vi "Message Loop Async.vi"(11 "OBS in":refnum<class "OBS.lvclass">) -> ()   [LabVIEW 2022 SP3, in "obs-websocket-lv.lvlib" / "OBS.lvclass"]
uses:
  OBS.lvclass
  State.ctl
  OBS.lvclass/OBS.ctl
  <vilib>/MediaMongrels Ltd/WebSockets/WebSockets/WebSocket Client/WebSocket Client.lvclass
panel:
  out "State":T1
  out "error IO":errorcluster
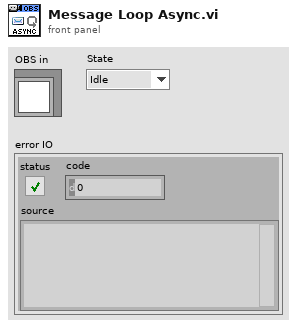
[diagram p1: front panel]
types:
  T1 = typedef "obs-websocket-lv.lvlib/OBS.lvclass/State.ctl" = enum16{"Idle", "Opening", "Open", "Closing", "Stopping"}
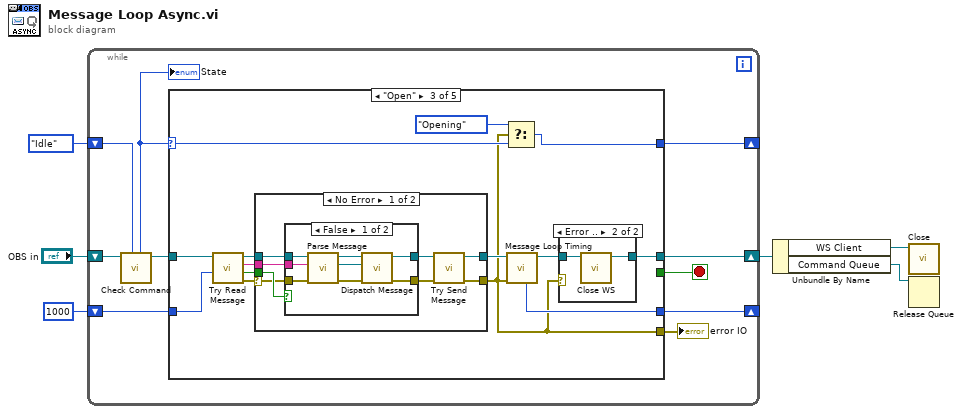
[diagram p0: block diagram]
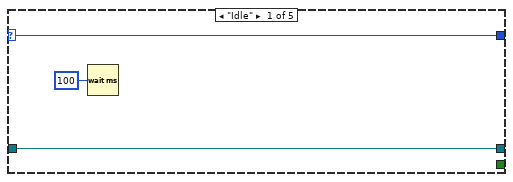
[diagram p2: hidden frame]
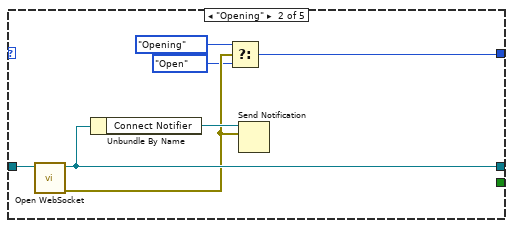
[diagram p3: hidden frame]
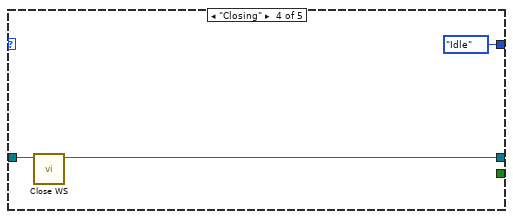
[diagram p7: hidden frame]
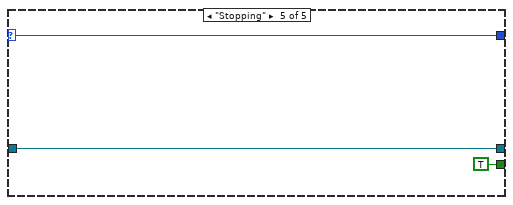
[diagram p8: hidden frame]
diagram:
  n1 = while {
    shift-right: [w12] -> _
    shift-left: 1000 -> [w13]
    shift-right: [w15] -> w5
    shift-left: "OBS in" -> [w11]
    shift-right: [w7] -> _
    shift-left: State."Idle" ("State") -> [w9]
    stop <- w16 stop-if-true
    n2 = call "Check Command.vi"("State"=w9, "OBS in"=w11) -> ("OBS out"=w10:refnum<class "OBS.lvclass">, "Next State"=w8:T1)  [unwired: 7 in, 1 out]
    "State" <- w8
    n3 = case shown="\"Open\"" w8 {
      selector: w8 -> [w18 _ w32 _ w67]
      tunnel: w10 -> [w19 w26 w40 w65 w68]
      tunnel: [_ _ _ _ TRUE ("Stop?")] -> w16
      tunnel: [w19 w24 w27 w64 w68] -> w15
      tunnel: [_ _ w28 _ _] -> w14
      tunnel: w13 -> [_ _ w34 _ _]
      tunnel: [_ _ w33 _ _] -> w12
      tunnel: [w18 w20 w30 State."Idle" ("State") w67] -> w7
      frame "Idle" {
        n4 = Wait (ms)(milliseconds to wait=u32 100) -> ()  [unwired: 1 out]
      }
      frame "Opening" {
        n5 = call "Open WebSocket.vi"("OBS in"=w26) -> ("error out"=w23:errorcluster, "OBS out"=w24:refnum<class "OBS.lvclass">)  [unwired: 9 in]
        n6 = Unbundle By Name(w24) -> ("Connect Notifier"=w25:refnum<notifier>)
        n7 = Select(t=State."Opening" ("State"), s=w23, f=State."Open" ("State")) -> (s? t:f=w20:T1)
        n8 = Send Notification(notification=w23, notifier=w25) -> ()  [unwired: 1 in, 2 out]
      }
      frame "Open" {
        n9 = call "Try Read Message.vi"("timeout ms (100)"=w34, "OBS in"=w40) -> ("error out"=w39:errorcluster, "Timeout"=w38:bool, "Data"=w37:string, "OBS out"=w36:refnum<class "OBS.lvclass">)  [unwired: 6 in]
        n10 = case shown="No Error" w39 {
          selector: w39 -> [w50 w63]
          tunnel: w38 -> [w51 _]
          tunnel: w37 -> [w49 _]
          tunnel: w36 -> [w48 w62]
          tunnel: [w45 w62] -> w35
          tunnel: [w44 w63] -> w28
          frame No Error {
            n11 = case shown="False" w51 {
              tunnel: w50 -> [w57 w60]
              tunnel: w49 -> [w58 _]
              tunnel: w48 -> [w59 w61]
              tunnel: [w53 w61] -> w47
              tunnel: [w52 w60] -> w46
              frame False {
                n12 = call "Parse Message.vi"("error in (no error)"=w57, "Data"=w58, "OBS in"=w59) -> ("error out"=w54:errorcluster, "Server Message"=w55:refnum<class "Server Message.lvclass">, "OBS out"=w56:refnum<class "OBS.lvclass">)  [unwired: 6 in]
                n13 = call "Dispatch Message.vi"("error in (no error)"=w54, "Server Message"=w55, "OBS in"=w56) -> ("error out"=w52:errorcluster, "OBS out"=w53:refnum<class "OBS.lvclass">)  [unwired: 7 in]
              }
              frame True {
              }
            }
            n14 = call "Try Send Message.vi"("error in (no error)"=w46, "OBS in"=w47) -> ("error out"=w44:errorcluster, "OBS out"=w45:refnum<class "OBS.lvclass">)  [unwired: 8 in]
          }
          frame Error {
          }
        }
        n15 = Select(t=State."Opening", s=w28, f=w32) -> (s? t:f=w30:T1)
        n16 = call "Message Loop Timing.vi"("error in (no error)"=w28, "OBS in"=w35) -> ("OBS out"=w29:refnum<class "OBS.lvclass">, "Next Timeout"=w33:i32)  [unwired: 7 in, 1 out]
        n17 = case shown="Error .." w28 {
          tunnel: w29 -> [w41 w43]
          tunnel: [w41 w42] -> w27
          frame No Error {
          }
          frame Error {
            n18 = call "Close WS.vi"("OBS in"=w43) -> ("OBS out"=w42:refnum<class "OBS.lvclass">)  [unwired: 9 in, 1 out]
          }
        }
      }
      frame "Closing" {
        n19 = call "Close WS.vi"("OBS in"=w65) -> ("OBS out"=w64:refnum<class "OBS.lvclass">)  [unwired: 9 in, 1 out]
      }
      frame "Stopping" {
      }
    }
    "error IO" <- w14
  }
  n20 = Unbundle By Name(w5) -> ("WS Client"=w4:refnum<class "WebSocket Client.lvclass">, "Command Queue"=w1:refnum<queue>)
  n21 = call-dynamic "Close.vi"("WebSocket in"=w4) -> ()  [unwired: 10 in, 1 out]
  n22 = Release Queue(queue=w1) -> ()  [unwired: 2 in, 3 out]
